vi "Read FGV Data.vi"(11 "Station Action.lvclass In":refnum<class "Station Action.lvclass">) -> (3 "Station Action.lvclass Out":refnum<class "Station Action.lvclass">)   [LabVIEW 2019]
uses:
  Station Action.lvclass
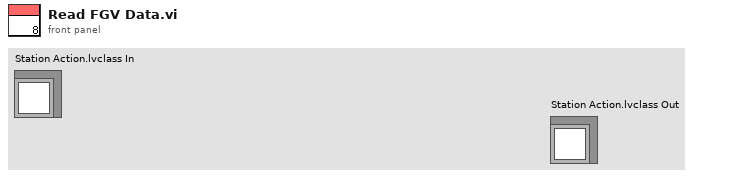
[diagram p1: front panel]
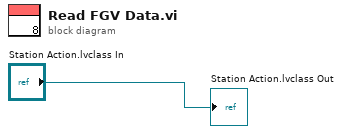
[diagram p0: block diagram]
diagram:
  "Station Action.lvclass Out" <- "Station Action.lvclass In"
